vi "Main.vi"(7 "sweep rate, /min":dbl=0.2, 8 "sweep to:":dbl=4.0, 9 "sweep":T8(radio)=enum."2636a_smub") -> ()   [LabVIEW 2021] (continued)
                        n662 = property on="data_caption" class="Str"("Value"=w727) -> ()  [unwired: 2 in, 2 out]
                      }
                      frame #26 {
                        # "measure time"
                        n663 = local read "measure time"() -> (w747:bool)
                        n664 = property on="Figure_axis" class="Arr (strict)"() -> ("Value"=w744:string[])  [unwired: 2 in, 2 out]
                        n665 = property on="data_caption" class="Str"() -> ("Value"=w746:string)  [unwired: 2 in, 2 out]
                        n666 = case shown="True" w747 {
                          tunnel: w746 -> [w749 w755]
                          tunnel: [w749 w754] -> w745
                          tunnel: w744 -> [w748 w752]
                          tunnel: [w748 w750] -> w743
                          frame False {
                            # "not measuring time"
                          }
                          frame True {
                            w751 = "time"
                            # "measuring time"
                            n667 = Build Array (concatenate)(w752, w751) -> (w750:string[])
                            n668 = Concatenate Strings(w755, w751, "\t") -> (w754:string)
                          }
                        }
                        n669 = property on="Figure_axis" class="Arr (strict)"("Value"=w743) -> ()  [unwired: 2 in, 2 out]
                        n670 = property on="data_caption" class="Str"("Value"=w745) -> ()  [unwired: 2 in, 2 out]
                      }
                      frame #27 {
                        # "Measure magnetic field on Teslatron_iPS"
                        n671 = local read "MagnetField"() -> (w760:bool)
                        n672 = property on="Figure_axis" class="Arr (strict)"() -> ("Value"=w757:string[])  [unwired: 2 in, 2 out]
                        n673 = property on="data_caption" class="Str"() -> ("Value"=w759:string)  [unwired: 2 in, 2 out]
                        n674 = case shown="True" w760 {
                          tunnel: w759 -> [w762 w768]
                          tunnel: [w762 w767] -> w758
                          tunnel: w757 -> [w761 w765]
                          tunnel: [w761 w763] -> w756
                          frame False {
                            # "do not Measure magnetic field on IPS120-0"
                          }
                          frame True {
                            w764 = "MagnetField"
                            # "Measure magnetic field on Teslatron_iPS_Field"
                            n675 = Build Array (concatenate)(w765, w764) -> (w763:string[])
                            n676 = Concatenate Strings(w768, w764, "\t") -> (w767:string)
                          }
                        }
                        n677 = property on="Figure_axis" class="Arr (strict)"("Value"=w756) -> ()  [unwired: 2 in, 2 out]
                        n678 = property on="data_caption" class="Str"("Value"=w758) -> ()  [unwired: 2 in, 2 out]
                      }
                      frame #28 {
                        # "Measure magnetic Temp on Teslatron_iPS"
                        n679 = property on="Magnet_T" class="Bool (strict)"() -> ("Value"=w769:bool)  [unwired: 2 in, 2 out]
                        n680 = property on="Figure_axis" class="Arr (strict)"() -> ("Value"=w771:string[])  [unwired: 2 in, 2 out]
                        n681 = property on="data_caption" class="Str"() -> ("Value"=w773:string)  [unwired: 2 in, 2 out]
                        n682 = case shown="True" w769 {
                          tunnel: w773 -> [w775 w781]
                          tunnel: [w775 w780] -> w772
                          tunnel: w771 -> [w774 w778]
                          tunnel: [w774 w776] -> w770
                          frame False {
                            # "do not Measure magnetic field on IPS120-0"
                          }
                          frame True {
                            w777 = "Magnet_Temp"
                            # "Measure magnetic field on Teslatron_iPS_Field"
                            n683 = Build Array (concatenate)(w778, w777) -> (w776:string[])
                            n684 = Concatenate Strings(w781, w777, "\t") -> (w780:string)
                          }
                        }
                        n685 = property on="Figure_axis" class="Arr (strict)"("Value"=w770) -> ()  [unwired: 2 in, 2 out]
                        n686 = property on="data_caption" class="Str"("Value"=w772) -> ()  [unwired: 2 in, 2 out]
                      }
                      frame #29 {
                        # "Measure SH_T on Teslatron_iPS"
                        n687 = property on="PT1" class="Bool (strict)"() -> ("Value"=w782:bool)  [unwired: 2 in, 2 out]
                        n688 = property on="Figure_axis" class="Arr (strict)"() -> ("Value"=w784:string[])  [unwired: 2 in, 2 out]
                        n689 = property on="data_caption" class="Str"() -> ("Value"=w786:string)  [unwired: 2 in, 2 out]
                        n690 = case shown="True" w782 {
                          tunnel: w786 -> [w788 w794]
                          tunnel: [w788 w793] -> w785
                          tunnel: w784 -> [w787 w791]
                          tunnel: [w787 w789] -> w783
                          frame False {
                            # "do not Measure magnetic field on IPS120-0"
                          }
                          frame True {
                            w790 = "PT1_Temp"
                            # "Measure magnetic field on Teslatron_iPS_Field"
                            n691 = Build Array (concatenate)(w791, w790) -> (w789:string[])
                            n692 = Concatenate Strings(w794, w790, "\t") -> (w793:string)
                          }
                        }
                        n693 = property on="Figure_axis" class="Arr (strict)"("Value"=w783) -> ()  [unwired: 2 in, 2 out]
                        n694 = property on="data_caption" class="Str"("Value"=w785) -> ()  [unwired: 2 in, 2 out]
                      }
                      frame #30 {
                        # "Measure magnetic field on Teslatron_iPS"
                        n695 = property on="MC_RuO2" class="Bool (strict)"() -> ("Value"=w795:bool)  [unwired: 2 in, 2 out]
                        n696 = property on="Figure_axis" class="Arr (strict)"() -> ("Value"=w797:string[])  [unwired: 2 in, 2 out]
                        n697 = property on="data_caption" class="Str"() -> ("Value"=w799:string)  [unwired: 2 in, 2 out]
                        n698 = case shown="True" w795 {
                          tunnel: w799 -> [w801 w807]
                          tunnel: [w801 w806] -> w798
                          tunnel: w797 -> [w800 w804]
                          tunnel: [w800 w802] -> w796
                          frame False {
                            # "not measure 2461 voltage (2461_meas_v)"
                          }
                          frame True {
                            w803 = "MC_RuO2_Temp"
                            n699 = Build Array (concatenate)(w804, w803) -> (w802:string[])
                            n700 = Concatenate Strings(w807, w803, "\t") -> (w806:string)
                          }
                        }
                        n701 = property on="Figure_axis" class="Arr (strict)"("Value"=w796) -> ()  [unwired: 2 in, 2 out]
                        n702 = property on="data_caption" class="Str"("Value"=w798) -> ()  [unwired: 2 in, 2 out]
                      }
                      frame #31 {
                        # "Measure magnetic field on Teslatron_iPS"
                        n703 = property on="Still" class="Bool (strict)"() -> ("Value"=w808:bool)  [unwired: 2 in, 2 out]
                        n704 = property on="Figure_axis" class="Arr (strict)"() -> ("Value"=w810:string[])  [unwired: 2 in, 2 out]
                        n705 = property on="data_caption" class="Str"() -> ("Value"=w812:string)  [unwired: 2 in, 2 out]
                        n706 = case shown="True" w808 {
                          tunnel: w812 -> [w814 w820]
                          tunnel: [w814 w819] -> w811
                          tunnel: w810 -> [w813 w817]
                          tunnel: [w813 w815] -> w809
                          frame False {
                            # "not measure 2461 voltage (2461_meas_v)"
                          }
                          frame True {
                            w816 = "Still_Temp"
                            n707 = Build Array (concatenate)(w817, w816) -> (w815:string[])
                            n708 = Concatenate Strings(w820, w816, "\t") -> (w819:string)
                          }
                        }
                        n709 = property on="Figure_axis" class="Arr (strict)"("Value"=w809) -> ()  [unwired: 2 in, 2 out]
                        n710 = property on="data_caption" class="Str"("Value"=w811) -> ()  [unwired: 2 in, 2 out]
                      }
                      frame #32 {
                        # "Measure magnetic field on Teslatron_iPS"
                        n711 = property on="Cold_Plate" class="Bool (strict)"() -> ("Value"=w821:bool)  [unwired: 2 in, 2 out]
                        n712 = property on="Figure_axis" class="Arr (strict)"() -> ("Value"=w823:string[])  [unwired: 2 in, 2 out]
                        n713 = property on="data_caption" class="Str"() -> ("Value"=w825:string)  [unwired: 2 in, 2 out]
                        n714 = case shown="True" w821 {
                          tunnel: w825 -> [w827 w833]
                          tunnel: [w827 w832] -> w824
                          tunnel: w823 -> [w826 w830]
                          tunnel: [w826 w828] -> w822
                          frame False {
                            # "not measure 2461 voltage (2461_meas_v)"
                          }
                          frame True {
                            w829 = "Cold_Plate_Temp"
                            n715 = Build Array (concatenate)(w830, w829) -> (w828:string[])
                            n716 = Concatenate Strings(w833, w829, "\t") -> (w832:string)
                          }
                        }
                        n717 = property on="Figure_axis" class="Arr (strict)"("Value"=w822) -> ()  [unwired: 2 in, 2 out]
                        n718 = property on="data_caption" class="Str"("Value"=w824) -> ()  [unwired: 2 in, 2 out]
                      }
                      frame #33 {
                        # "Measure magnetic field on Teslatron_iPS"
                        n719 = property on="PT2" class="Bool (strict)"() -> ("Value"=w834:bool)  [unwired: 2 in, 2 out]
                        n720 = property on="Figure_axis" class="Arr (strict)"() -> ("Value"=w836:string[])  [unwired: 2 in, 2 out]
                        n721 = property on="data_caption" class="Str"() -> ("Value"=w838:string)  [unwired: 2 in, 2 out]
                        n722 = case shown="True" w834 {
                          tunnel: w838 -> [w840 w846]
                          tunnel: [w840 w845] -> w837
                          tunnel: w836 -> [w839 w843]
                          tunnel: [w839 w841] -> w835
                          frame False {
                            # "not measure 2461 voltage (2461_meas_v)"
                          }
                          frame True {
                            w842 = "PT2_Temp"
                            n723 = Build Array (concatenate)(w843, w842) -> (w841:string[])
                            n724 = Concatenate Strings(w846, w842, "\t") -> (w845:string)
                          }
                        }
                        n725 = property on="Figure_axis" class="Arr (strict)"("Value"=w835) -> ()  [unwired: 2 in, 2 out]
                        n726 = property on="data_caption" class="Str"("Value"=w837) -> ()  [unwired: 2 in, 2 out]
                      }
                      frame #34 {
                        # "Measure magnetic field on Teslatron_iPS"
                        n727 = property on="MC_Cernox" class="Bool (strict)"() -> ("Value"=w847:bool)  [unwired: 2 in, 2 out]
                        n728 = property on="Figure_axis" class="Arr (strict)"() -> ("Value"=w849:string[])  [unwired: 2 in, 2 out]
                        n729 = property on="data_caption" class="Str"() -> ("Value"=w851:string)  [unwired: 2 in, 2 out]
                        n730 = case shown="True" w847 {
                          tunnel: w851 -> [w853 w859]
                          tunnel: [w853 w858] -> w850
                          tunnel: w849 -> [w852 w856]
                          tunnel: [w852 w854] -> w848
                          frame False {
                            # "not measure 2461 voltage (2461_meas_v)"
                          }
                          frame True {
                            w855 = "MC_Cernox_Temp"
                            n731 = Build Array (concatenate)(w856, w855) -> (w854:string[])
                            n732 = Concatenate Strings(w859, w855, "\t") -> (w858:string)
                          }
                        }
                        n733 = property on="Figure_axis" class="Arr (strict)"("Value"=w848) -> ()  [unwired: 2 in, 2 out]
                        n734 = property on="data_caption" class="Str"("Value"=w850) -> ()  [unwired: 2 in, 2 out]
                      }
                      frame #35 {
                        # "Measure magnetic field on Teslatron_iPS"
                        n735 = property on="MFLI1_AuxOut0" class="Bool (strict)"() -> ("Value"=w860:bool)  [unwired: 2 in, 2 out]
                        n736 = property on="Figure_axis" class="Arr (strict)"() -> ("Value"=w862:string[])  [unwired: 2 in, 2 out]
                        n737 = property on="data_caption" class="Str"() -> ("Value"=w864:string)  [unwired: 2 in, 2 out]
                        n738 = case shown="True" w860 {
                          tunnel: w864 -> [w866 w872]
                          tunnel: [w866 w871] -> w863
                          tunnel: w862 -> [w865 w869]
                          tunnel: [w865 w867] -> w861
                          frame False {
                            # "not measure 2461 voltage (2461_meas_v)"
                          }
                          frame True {
                            w868 = "V_Sweep_AuxOut0"
                            n739 = Build Array (concatenate)(w869, w868) -> (w867:string[])
                            n740 = Concatenate Strings(w872, w868, "\t") -> (w871:string)
                          }
                        }
                        n741 = property on="Figure_axis" class="Arr (strict)"("Value"=w861) -> ()  [unwired: 2 in, 2 out]
                        n742 = property on="data_caption" class="Str"("Value"=w863) -> ()  [unwired: 2 in, 2 out]
                      }
                    }
                  }
                  frame #2 {
                    # "0 = SR830_1_ip\n1 = SR830_1_oop\n2 = SR830_2_ip\n3 = SR830_2_oop\n4 = SR830_3_ip\n5 = SR830_3_oop\n6 = SR830_4_ip \n7 = SR830_4_oop \n8 = SR830_5_ip \n9 = SR830_5_oop \n10= 2400_1_v \n11= 2400_1_i \n12 = 2400_2_v\n13 = 2400_2_i \n14 = 2400_3_v \n15 = 2400_3_i \n16 = 2182A_1_ch1 \n17 = 2182A_1_ch2 \n18 = 2182A_2_ch1 \n19 = 2182A_2_ch2\n20 = 2182A_3_ch1 \n21 = 2182A_3_ch2 \n22 = 2182A_4_ch1 \n23 = 2182A_4_ch2 \n24 = 2636A_smua_v \n25 = 2636A_smua_i \n26 = 2636A_smub_v \n27 = 2636A_smub_i \n28 = time\n29 = iPS_Field\n30 = iPS_Magnet_T\n31 = iPS__SH_T\n32 = iTC _sample_T\n33 = iTC _VTI_T\n34 = iTC _PT1_T\n35 = iTC _PT2_T\n36 = iTC _VTI_P\n37 = 2461_meas_v\n38= 2461_meas_i\n39= Step_Value\n40= HyperLoop_Step\n41= SuperHyper_Step"
                    n743 = stacked-sequence {
                      frame #0 {
                        w877 = dbl[] []  # Empty array for data
                        # "clear data array before each measurement cycle"
                        n744 = property on="data" class="Arr (strict)"("Value"=w877) -> (error out=w876:errorcluster)  [unwired: 2 in, 1 out]
                        n745 = property on="Sweep Channel" class="DigNum (strict)"() -> ("Value"=w873:dbl)  [unwired: 2 in, 2 out]
                        n746 = property on="data" class="Arr (strict)"(error in=w876) -> ("Value"=w875:dbl[])  [unwired: 1 in, 2 out]
                        n747 = Build Array (concatenate)(w875, w873) -> (w874:dbl[])
                        n748 = property on="data" class="Arr (strict)"("Value"=w874) -> ()  [unwired: 2 in, 2 out]
                      }
                      frame #1 {
                        n749 = stacked-sequence "measurement sequence" {
                          frame #0 {
                            # "check if in-phase\nsignal on lock-in 1 \nis to be measured"
                            n750 = property on="data" class="Arr (strict)"() -> ("Value"=w879:dbl[])  [unwired: 2 in, 2 out]
                            n751 = local read "SR830 1 ip"() -> (w878:bool)
                            n752 = case shown="True" w878 {
                              tunnel: w879 -> [w881 w890]
                              tunnel: [w881 w889] -> w880
                              frame False {
                                # "we are not measuring in phase signal on lock-in 1 (SR830_1_ip)"
                              }
                              frame True {
                                # "we are  measuring lock-in 1, in phase (SR830_1_ip)"
                                n753 = local read "SR830 1 addr"() -> (w883:u8)
                                n754 = Number To Decimal String(number=w883) -> (decimal integer string=w882:string)  [unwired: 1 in]
                                n755 = GPIB Write(0:w882, 1:"OUTR?1") -> (6:w888:errorcluster)  [unwired: 3 in, 1 out]
                                n756 = GPIB Read(0:w882, 1:3200, 3:w888) -> (5:w886:string)  [unwired: 2 in, 2 out]
                                n757 = Fract/Exp String To Number(string=w886) -> (number=w885:dbl)  [unwired: 3 in, 1 out]
                                n758 = Build Array (concatenate)(w890, w885) -> (w889:dbl[])
                              }
                            }
                            n759 = property on="data" class="Arr (strict)"("Value"=w880) -> ()  [unwired: 2 in, 2 out]
                          }
                          frame #1 {
                            # "check if out-of-phase\nsignal on lock-in 1 \nis to be measured"
                            n760 = property on="data" class="Arr (strict)"() -> ("Value"=w892:dbl[])  [unwired: 2 in, 2 out]
                            n761 = local read "SR830 1 oop"() -> (w891:bool)
                            n762 = case shown="True" w891 {
                              tunnel: w892 -> [w894 w903]
                              tunnel: [w894 w902] -> w893
                              frame False {
                                # "we are not measuring out of phase signal on lock-in 1 (SR830_1_oop)"
                              }
                              frame True {
                                # "we are  measuring lock-in 1, out of phase (SR830_1_oop)"
                                n763 = local read "SR830 1 addr"() -> (w896:u8)
                                n764 = Number To Decimal String(number=w896) -> (decimal integer string=w895:string)  [unwired: 1 in]
                                n765 = GPIB Write(0:w895, 1:"OUTR?2") -> (6:w901:errorcluster)  [unwired: 3 in, 1 out]
                                n766 = GPIB Read(0:w895, 1:3200, 3:w901) -> (5:w899:string)  [unwired: 2 in, 2 out]
                                n767 = Fract/Exp String To Number(string=w899) -> (number=w898:dbl)  [unwired: 3 in, 1 out]
                                n768 = Build Array (concatenate)(w903, w898) -> (w902:dbl[])
                              }
                            }
                            n769 = property on="data" class="Arr (strict)"("Value"=w893) -> ()  [unwired: 2 in, 2 out]
                          }
                          frame #2 {
                            # "check if in-phase\nsignal on lock-in 2 \nis to be measured"
                            n770 = property on="data" class="Arr (strict)"() -> ("Value"=w905:dbl[])  [unwired: 2 in, 2 out]
                            n771 = local read "SR830 2 ip"() -> (w904:bool)
                            n772 = case shown="True" w904 {
                              tunnel: w905 -> [w907 w916]
                              tunnel: [w907 w915] -> w906
                              frame False {
                                # "we are not measuring in phase signal on lock-in 2 (SR830_2_ip)"
                              }
                              frame True {
                                # "we are  measuring lock-in 2, in phase (SR830_2_ip)"
                                n773 = local read "SR830 2 addr"() -> (w909:u8)
                                n774 = Number To Decimal String(number=w909) -> (decimal integer string=w908:string)  [unwired: 1 in]
                                n775 = GPIB Write(0:w908, 1:"OUTP?1") -> (6:w914:errorcluster)  [unwired: 3 in, 1 out]
                                n776 = GPIB Read(0:w908, 1:3200, 3:w914) -> (5:w912:string)  [unwired: 2 in, 2 out]
                                n777 = Fract/Exp String To Number(string=w912) -> (number=w911:dbl)  [unwired: 3 in, 1 out]
                                n778 = Build Array (concatenate)(w916, w911) -> (w915:dbl[])
                              }
                            }
                            n779 = property on="data" class="Arr (strict)"("Value"=w906) -> ()  [unwired: 2 in, 2 out]
                          }
                          frame #3 {
                            # "check if out-of-phase\nsignal on lock-in 2 \nis to be measured"
                            n780 = property on="data" class="Arr (strict)"() -> ("Value"=w918:dbl[])  [unwired: 2 in, 2 out]
                            n781 = local read "SR830 2 oop"() -> (w917:bool)
                            n782 = case shown="True" w917 {
                              tunnel: w918 -> [w920 w929]
                              tunnel: [w920 w928] -> w919
                              frame False {
                                # "we are not measuring out of phase signal on lock-in 2 (SR830_2_oop)"
                              }
                              frame True {
                                # "we are  measuring lock-in 2, out of phase (SR830_2_oop)"
                                n783 = local read "SR830 2 addr"() -> (w922:u8)
                                n784 = Number To Decimal String(number=w922) -> (decimal integer string=w921:string)  [unwired: 1 in]
                                n785 = GPIB Write(0:w921, 1:"OUTP?2") -> (6:w927:errorcluster)  [unwired: 3 in, 1 out]
                                n786 = GPIB Read(0:w921, 1:3200, 3:w927) -> (5:w925:string)  [unwired: 2 in, 2 out]
                                n787 = Fract/Exp String To Number(string=w925) -> (number=w924:dbl)  [unwired: 3 in, 1 out]
                                n788 = Build Array (concatenate)(w929, w924) -> (w928:dbl[])
                              }
                            }
                            n789 = property on="data" class="Arr (strict)"("Value"=w919) -> ()  [unwired: 2 in, 2 out]
                          }
                          frame #4 {
                            # "check if in-phase\nsignal on lock-in 3 \nis to be measured"
                            n790 = property on="data" class="Arr (strict)"() -> ("Value"=w931:dbl[])  [unwired: 2 in, 2 out]
                            n791 = local read "SR830 3 ip"() -> (w930:bool)
                            n792 = case shown="True" w930 {
                              tunnel: w931 -> [w933 w942]
                              tunnel: [w933 w941] -> w932
                              frame False {
                                # "we are not measuring in phase signal on lock-in 3 (SR830_3_ip)"
                              }
                              frame True {
                                # "we are  measuring lock-in 3, in phase (SR830_3_ip)"
                                n793 = local read "SR830 3 addr"() -> (w935:u8)
                                n794 = Number To Decimal String(number=w935) -> (decimal integer string=w934:string)  [unwired: 1 in]
                                n795 = GPIB Write(0:w934, 1:"OUTP?1") -> (6:w940:errorcluster)  [unwired: 3 in, 1 out]
                                n796 = GPIB Read(0:w934, 1:3200, 3:w940) -> (5:w938:string)  [unwired: 2 in, 2 out]
                                n797 = Fract/Exp String To Number(string=w938) -> (number=w937:dbl)  [unwired: 3 in, 1 out]
                                n798 = Build Array (concatenate)(w942, w937) -> (w941:dbl[])
                              }
                            }
                            n799 = property on="data" class="Arr (strict)"("Value"=w932) -> ()  [unwired: 2 in, 2 out]
                          }
                          frame #5 {
                            # "check if out-of-phase\nsignal on lock-in 3 \nis to be measured"
                            n800 = property on="data" class="Arr (strict)"() -> ("Value"=w944:dbl[])  [unwired: 2 in, 2 out]
                            n801 = local read "SR830 3 oop"() -> (w943:bool)
                            n802 = case shown="True" w943 {
                              tunnel: w944 -> [w946 w955]
                              tunnel: [w946 w954] -> w945
                              frame False {
                                # "we are not measuring out of phase signal on lock-in 3 (SR830_3_oop)"
                              }
                              frame True {
                                # "we are  measuring lock-in 3, out of phase (SR830_3_oop)"
                                n803 = local read "SR830 3 addr"() -> (w948:u8)
                                n804 = Number To Decimal String(number=w948) -> (decimal integer string=w947:string)  [unwired: 1 in]
                                n805 = GPIB Write(0:w947, 1:"OUTP?2") -> (6:w953:errorcluster)  [unwired: 3 in, 1 out]
                                n806 = GPIB Read(0:w947, 1:3200, 3:w953) -> (5:w951:string)  [unwired: 2 in, 2 out]
                                n807 = Fract/Exp String To Number(string=w951) -> (number=w950:dbl)  [unwired: 3 in, 1 out]
                                n808 = Build Array (concatenate)(w955, w950) -> (w954:dbl[])
                              }
                            }
                            n809 = property on="data" class="Arr (strict)"("Value"=w945) -> ()  [unwired: 2 in, 2 out]
                          }
                          frame #6 {
                            # "check if in-phase\nsignal on lock-in 4 \nis to be measured"
                            n810 = property on="data" class="Arr (strict)"() -> ("Value"=w957:dbl[])  [unwired: 2 in, 2 out]
                            n811 = local read "SR830 4 ip"() -> (w956:bool)
                            n812 = case shown="True" w956 {
                              tunnel: w957 -> [w959 w968]
                              tunnel: [w959 w967] -> w958
                              frame False {
                                # "we are not measuring in phase signal on lock-in 4 (SR830_4_ip)"
                              }
                              frame True {
                                # "we are  measuring lock-in 4, in phase (SR830_4_ip)"
                                n813 = local read "SR830 4 addr"() -> (w961:u8)
                                n814 = Number To Decimal String(number=w961) -> (decimal integer string=w960:string)  [unwired: 1 in]
                                n815 = GPIB Write(0:w960, 1:"OUTP?1") -> (6:w966:errorcluster)  [unwired: 3 in, 1 out]
                                n816 = GPIB Read(0:w960, 1:3200, 3:w966) -> (5:w964:string)  [unwired: 2 in, 2 out]
                                n817 = Fract/Exp String To Number(string=w964) -> (number=w963:dbl)  [unwired: 3 in, 1 out]
                                n818 = Build Array (concatenate)(w968, w963) -> (w967:dbl[])
                              }
                            }
                            n819 = property on="data" class="Arr (strict)"("Value"=w958) -> ()  [unwired: 2 in, 2 out]
                          }
                          frame #7 {
                            # "check if out-of-phase\nsignal on lock-in 4 \nis to be measured"
                            n820 = property on="data" class="Arr (strict)"() -> ("Value"=w970:dbl[])  [unwired: 2 in, 2 out]
                            n821 = local read "SR830 4 oop"() -> (w969:bool)
                            n822 = case shown="True" w969 {
                              tunnel: w970 -> [w972 w981]
                              tunnel: [w972 w980] -> w971
                              frame False {
                                # "we are not measuring out of phase signal on lock-in 4 (SR830_4_oop)"
                              }
                              frame True {
                                # "we are  measuring lock-in 4, out of phase (SR830_4_oop)"
                                n823 = local read "SR830 4 addr"() -> (w974:u8)
                                n824 = Number To Decimal String(number=w974) -> (decimal integer string=w973:string)  [unwired: 1 in]
                                n825 = GPIB Write(0:w973, 1:"OUTP?2") -> (6:w979:errorcluster)  [unwired: 3 in, 1 out]
                                n826 = GPIB Read(0:w973, 1:3200, 3:w979) -> (5:w977:string)  [unwired: 2 in, 2 out]
                                n827 = Fract/Exp String To Number(string=w977) -> (number=w976:dbl)  [unwired: 3 in, 1 out]
                                n828 = Build Array (concatenate)(w981, w976) -> (w980:dbl[])
                              }
                            }
                            n829 = property on="data" class="Arr (strict)"("Value"=w971) -> ()  [unwired: 2 in, 2 out]
                          }
                          frame #8 {
                            n830 = property on="data" class="Arr (strict)"() -> ("Value"=w983:dbl[])  [unwired: 2 in, 2 out]
                            n831 = local read "SR830 5 ip"() -> (w982:bool)
                            n832 = case shown="True" w982 {
                              tunnel: w983 -> [w985 w994]
                              tunnel: [w985 w993] -> w984
                              frame False {
                              }
                              frame True {
                                n833 = local read "SR830 5 addr"() -> (w987:u8)
                                n834 = Number To Decimal String(number=w987) -> (decimal integer string=w986:string)  [unwired: 1 in]
                                n835 = GPIB Write(0:w986, 1:"OUTP?1") -> (6:w992:errorcluster)  [unwired: 3 in, 1 out]
                                n836 = GPIB Read(0:w986, 1:3200, 3:w992) -> (5:w990:string)  [unwired: 2 in, 2 out]
                                n837 = Fract/Exp String To Number(string=w990) -> (number=w989:dbl)  [unwired: 3 in, 1 out]
                                n838 = Build Array (concatenate)(w994, w989) -> (w993:dbl[])
                              }
                            }
                            n839 = property on="data" class="Arr (strict)"("Value"=w984) -> ()  [unwired: 2 in, 2 out]
                          }
                          frame #9 {
                            n840 = property on="data" class="Arr (strict)"() -> ("Value"=w996:dbl[])  [unwired: 2 in, 2 out]
                            n841 = local read "SR830 5 oop"() -> (w995:bool)
                            n842 = case shown="True" w995 {
                              tunnel: w996 -> [w998 w1007]
                              tunnel: [w998 w1006] -> w997
                              frame False {
                                # "we are not measuring out of phase signal on lock-in 4 (SR830_4_oop)"
                              }
                              frame True {
                                n843 = local read "SR830 5 addr"() -> (w1000:u8)
                                n844 = Number To Decimal String(number=w1000) -> (decimal integer string=w999:string)  [unwired: 1 in]
                                n845 = GPIB Write(0:w999, 1:"OUTP?2") -> (6:w1005:errorcluster)  [unwired: 3 in, 1 out]
                                n846 = GPIB Read(0:w999, 1:3200, 3:w1005) -> (5:w1003:string)  [unwired: 2 in, 2 out]
                                n847 = Fract/Exp String To Number(string=w1003) -> (number=w1002:dbl)  [unwired: 3 in, 1 out]
                                n848 = Build Array (concatenate)(w1007, w1002) -> (w1006:dbl[])
                              }
                            }
                            n849 = property on="data" class="Arr (strict)"("Value"=w997) -> ()  [unwired: 2 in, 2 out]
                          }
                          frame #10 {
                            # "check if voltage \non 2400 SouceMeter 1\nis to be measured"
                            n850 = property on="data" class="Arr (strict)"() -> ("Value"=w1009:dbl[])  [unwired: 2 in, 2 out]
                            n851 = local read "2400 1 meas v"() -> (w1008:bool)
                            n852 = case shown="True" w1008 {
                              tunnel: w1009 -> [w1011 w1022]
                              tunnel: [w1011 w1021] -> w1010
                              frame False {
                                # "we are not measuring 2400 1, voltage (2400_1_v)"
                              }
                              frame True {
                                # "we are  measuring 2400 1, voltage (2400_1_v)"
                                n853 = local read "2400 1 addr"() -> (w1016:u8)
                                n854 = Number To Decimal String(number=w1016) -> (decimal integer string=w1015:string)  [unwired: 1 in]
                                n855 = GPIB Write(0:w1015, 1:":READ?") -> (6:w1020:errorcluster)  [unwired: 3 in, 1 out]
                                n856 = GPIB Read(0:w1015, 1:3200, 3:w1020) -> (5:w1013:string)  [unwired: 2 in, 2 out]
                                n857 = String Subset(string=w1013, length (rest)=13) -> (substring=w1012:string)  [unwired: 1 in]
                                n858 = Fract/Exp String To Number(string=w1012) -> (number=w1018:dbl)  [unwired: 3 in, 1 out]
                                n859 = Build Array (concatenate)(w1022, w1018) -> (w1021:dbl[])
                              }
                            }
                            n860 = property on="data" class="Arr (strict)"("Value"=w1010) -> ()  [unwired: 2 in, 2 out]
                          }
                          frame #11 {
                            # "check if current \non 2400 SouceMeter 1\nis to be measured"
                            n861 = property on="data" class="Arr (strict)"() -> ("Value"=w1024:dbl[])  [unwired: 2 in, 2 out]
                            n862 = local read "2400 1 meas i"() -> (w1023:bool)
                            n863 = case shown="True" w1023 {
                              tunnel: w1024 -> [w1026 w1038]
                              tunnel: [w1026 w1037] -> w1025
                              frame False {
                                # "we are not measuring 2400 1, current (2400_1_i)"
                              }
                              frame True {
                                # "we are  measuring 2400 1, current (2400_1_i)"
                                n864 = local read "2400 1 addr"() -> (w1032:u8)
                                n865 = Number To Decimal String(number=w1032) -> (decimal integer string=w1031:string)  [unwired: 1 in]
                                n866 = GPIB Write(0:w1031, 1:":READ?") -> (6:w1036:errorcluster)  [unwired: 3 in, 1 out]
                                n867 = GPIB Read(0:w1031, 1:3200, 3:w1036) -> (5:w1029:string)  [unwired: 2 in, 2 out]
                                n868 = String Subset(string=w1029, offset (0)=14, length (rest)=13) -> (substring=w1028:string)
                                n869 = Fract/Exp String To Number(string=w1028) -> (number=w1034:dbl)  [unwired: 3 in, 1 out]
                                n870 = Build Array (concatenate)(w1038, w1034) -> (w1037:dbl[])
                              }
                            }
                            n871 = property on="data" class="Arr (strict)"("Value"=w1025) -> ()  [unwired: 2 in, 2 out]
                          }
                          frame #12 {
                            # "check if voltage \non 2400 SouceMeter 2\nis to be measured"
                            n872 = property on="data" class="Arr (strict)"() -> ("Value"=w1040:dbl[])  [unwired: 2 in, 2 out]
                            n873 = local read "2400 2 meas v"() -> (w1039:bool)
                            n874 = case shown="True" w1039 {
                              tunnel: w1040 -> [w1042 w1053]
                              tunnel: [w1042 w1052] -> w1041
                              frame False {
                                # "we are not measuring 2400 2, voltage (2400_2_v)"
                              }
                              frame True {
                                # "we are  measuring 2400 2, voltage (2400_2_v)"
                                n875 = local read "2400 2 addr"() -> (w1047:u8)
                                n876 = Number To Decimal String(number=w1047) -> (decimal integer string=w1046:string)  [unwired: 1 in]
                                n877 = GPIB Write(0:w1046, 1:":READ?") -> (6:w1051:errorcluster)  [unwired: 3 in, 1 out]
                                n878 = GPIB Read(0:w1046, 1:3200, 3:w1051) -> (5:w1044:string)  [unwired: 2 in, 2 out]
                                n879 = String Subset(string=w1044, length (rest)=13) -> (substring=w1043:string)  [unwired: 1 in]
                                n880 = Fract/Exp String To Number(string=w1043) -> (number=w1049:dbl)  [unwired: 3 in, 1 out]
                                n881 = Build Array (concatenate)(w1053, w1049) -> (w1052:dbl[])
                              }
                            }
                            n882 = property on="data" class="Arr (strict)"("Value"=w1041) -> ()  [unwired: 2 in, 2 out]
                          }
                          frame #13 {
                            # "check if current \non 2400 SouceMeter 2\nis to be measured"
                            n883 = property on="data" class="Arr (strict)"() -> ("Value"=w1055:dbl[])  [unwired: 2 in, 2 out]
                            n884 = local read "2400 2 meas i"() -> (w1054:bool)
                            n885 = case shown="True" w1054 {
                              tunnel: w1055 -> [w1057 w1069]
                              tunnel: [w1057 w1068] -> w1056
                              frame False {
                                # "we are not measuring 2400 2, current (2400_2_i)"
                              }
                              frame True {
                                # "we are  measuring 2400 2, current (2400_2_i)"
                                n886 = local read "2400 2 addr"() -> (w1063:u8)
                                n887 = Number To Decimal String(number=w1063) -> (decimal integer string=w1062:string)  [unwired: 1 in]
                                n888 = GPIB Write(0:w1062, 1:":READ?") -> (6:w1067:errorcluster)  [unwired: 3 in, 1 out]
                                n889 = GPIB Read(0:w1062, 1:3200, 3:w1067) -> (5:w1060:string)  [unwired: 2 in, 2 out]
                                n890 = String Subset(string=w1060, offset (0)=14, length (rest)=13) -> (substring=w1059:string)
                                n891 = Fract/Exp String To Number(string=w1059) -> (number=w1065:dbl)  [unwired: 3 in, 1 out]
                                n892 = Build Array (concatenate)(w1069, w1065) -> (w1068:dbl[])
                              }
                            }
                            n893 = property on="data" class="Arr (strict)"("Value"=w1056) -> ()  [unwired: 2 in, 2 out]
                          }
                          frame #14 {
                            # "check if voltage \non 2400 SouceMeter 3\nis to be measured"
                            n894 = property on="data" class="Arr (strict)"() -> ("Value"=w1071:dbl[])  [unwired: 2 in, 2 out]
                            n895 = local read "2400 3 meas v"() -> (w1070:bool)
                            n896 = case shown="True" w1070 {
                              tunnel: w1071 -> [w1073 w1084]
                              tunnel: [w1073 w1083] -> w1072
                              frame False {
                                # "we are not measuring 2400 3, voltage (2400_3_v)"
                              }
                              frame True {
                                # "we are  measuring 2400 3, voltage (2400_3_v)"
                                n897 = local read "2400 3 addr"() -> (w1078:u8)
                                n898 = Number To Decimal String(number=w1078) -> (decimal integer string=w1077:string)  [unwired: 1 in]
                                n899 = GPIB Write(0:w1077, 1:":READ?") -> (6:w1082:errorcluster)  [unwired: 3 in, 1 out]
                                n900 = GPIB Read(0:w1077, 1:3200, 3:w1082) -> (5:w1075:string)  [unwired: 2 in, 2 out]
                                n901 = String Subset(string=w1075, length (rest)=13) -> (substring=w1074:string)  [unwired: 1 in]
                                n902 = Fract/Exp String To Number(string=w1074) -> (number=w1080:dbl)  [unwired: 3 in, 1 out]
                                n903 = Build Array (concatenate)(w1084, w1080) -> (w1083:dbl[])
                              }
                            }
                            n904 = property on="data" class="Arr (strict)"("Value"=w1072) -> ()  [unwired: 2 in, 2 out]
                          }
                          frame #15 {
                            # "check if current \non 2400 SouceMeter 3\nis to be measured"
                            n905 = property on="data" class="Arr (strict)"() -> ("Value"=w1086:dbl[])  [unwired: 2 in, 2 out]
                            n906 = local read "2400 3 meas i"() -> (w1085:bool)
                            n907 = case shown="True" w1085 {
                              tunnel: w1086 -> [w1088 w1100]
                              tunnel: [w1088 w1099] -> w1087
                              frame False {
                                # "we are not measuring 2400 3, current (2400_3_i)"
                              }
                              frame True {
                                # "we are  measuring 2400 3, current (2400_3_i)"
                                n908 = local read "2400 3 addr"() -> (w1094:u8)
                                n909 = Number To Decimal String(number=w1094) -> (decimal integer string=w1093:string)  [unwired: 1 in]
                                n910 = GPIB Write(0:w1093, 1:":READ?") -> (6:w1098:errorcluster)  [unwired: 3 in, 1 out]
                                n911 = GPIB Read(0:w1093, 1:3200, 3:w1098) -> (5:w1091:string)  [unwired: 2 in, 2 out]
                                n912 = String Subset(string=w1091, offset (0)=14, length (rest)=13) -> (substring=w1090:string)
                                n913 = Fract/Exp String To Number(string=w1090) -> (number=w1096:dbl)  [unwired: 3 in, 1 out]
                                n914 = Build Array (concatenate)(w1100, w1096) -> (w1099:dbl[])
                              }
                            }
                            n915 = property on="data" class="Arr (strict)"("Value"=w1087) -> ()  [unwired: 2 in, 2 out]
                          }
                          frame #16 {
                            # "check if 1st channel \non Keithley 2182A 1\nis to be measured"
                            n916 = property on="data" class="Arr (strict)"() -> ("Value"=w1102:dbl[])  [unwired: 2 in, 2 out]
                            n917 = local read "2182A 1 ch1"() -> (w1101:bool)
                            n918 = case shown="True" w1101 {
                              tunnel: w1102 -> [w1104 w1113]
                              tunnel: [w1104 w1112] -> w1103
                              frame False {
                                # "we are not measuring 2182A 1 channel 1 (2182A_1_ch1)"
                              }
                              frame True {
                                # "we are  measuring 2182A 1 channel 1 (2182A_1_ch1)"
                                n919 = local read "2182A 1 addr"() -> (w1107:u8)
                                n920 = Number To Decimal String(number=w1107) -> (decimal integer string=w1106:string)  [unwired: 1 in]
                                n921 = GPIB Write(0:w1106, 1:":SENSe:DATA:FRES?") -> (6:w1111:errorcluster)  [unwired: 3 in, 1 out]
                                n922 = GPIB Read(0:w1106, 1:200, 3:w1111) -> (5:w1105:string)  [unwired: 2 in, 2 out]
                                n923 = Fract/Exp String To Number(string=w1105) -> (number=w1109:dbl)  [unwired: 3 in, 1 out]
                                n924 = Build Array (concatenate)(w1113, w1109) -> (w1112:dbl[])
                              }
                            }
                            n925 = property on="data" class="Arr (strict)"("Value"=w1103) -> ()  [unwired: 2 in, 2 out]
                          }
                          frame #17 {
                            # "check if 2nd channel \non Keithley 2182A 1\nis to be measured"
                            n926 = property on="data" class="Arr (strict)"() -> ("Value"=w1115:dbl[])  [unwired: 2 in, 2 out]
                            n927 = local read "2182A 1 ch2"() -> (w1114:bool)
                            n928 = case shown="True" w1114 {
                              tunnel: w1115 -> [w1117 w1130]
                              tunnel: [w1117 w1129] -> w1116
                              frame False {
                                # "we are not measuring 2182A 1 channel 2 (2182A_1_ch2)"
                              }
                              frame True {
                                # "switching to channel 2 and then\nback to channel 1"
                                # "we are  measuring 2182A 1 channel 2 (2182A_1_ch2)"
                                n929 = local read "2182A 1 addr"() -> (w1124:u8)
                                n930 = Number To Decimal String(number=w1124) -> (decimal integer string=w1119:string)  [unwired: 1 in]
                                n931 = GPIB Write(0:w1119, 1:":SENSe:CHAN 2") -> (6:w1121:errorcluster)  [unwired: 3 in, 1 out]
                                n932 = GPIB Write(0:w1119, 1:":SENSe:DATA:FRES?", 3:w1121) -> (6:w1128:errorcluster)  [unwired: 2 in, 1 out]
                                n933 = GPIB Read(0:w1119, 1:200, 3:w1128) -> (5:w1123:string, 7:w1120:errorcluster)  [unwired: 2 in, 1 out]
                                n934 = GPIB Write(0:w1119, 1:":SENSe:CHAN 1", 3:w1120) -> ()  [unwired: 2 in, 2 out]
                                n935 = Fract/Exp String To Number(string=w1123) -> (number=w1126:dbl)  [unwired: 3 in, 1 out]
                                n936 = Build Array (concatenate)(w1130, w1126) -> (w1129:dbl[])
                              }
                            }
                            n937 = property on="data" class="Arr (strict)"("Value"=w1116) -> ()  [unwired: 2 in, 2 out]
                          }
                          frame #18 {
                            # "check if 1st channel \non Keithley 2182A 2\nis to be measured"
                            n938 = property on="data" class="Arr (strict)"() -> ("Value"=w1132:dbl[])  [unwired: 2 in, 2 out]
                            n939 = local read "2182A 2 ch1"() -> (w1131:bool)
                            n940 = case shown="False" w1131 {
                              tunnel: w1132 -> [w1134 w1143]
                              tunnel: [w1134 w1142] -> w1133
                              frame False {
                                # "we are not measuring 2182A 2 channel 1 (2182A_2_ch1)"
                              }
                              frame True {
                                # "we are  measuring 2182A 2 channel 1 (2182A_2_ch1)"
                                n941 = local read "2182A 2 addr"() -> (w1137:u8)
                                n942 = Number To Decimal String(number=w1137) -> (decimal integer string=w1136:string)  [unwired: 1 in]
                                n943 = GPIB Write(0:w1136, 1:":SENSe:DATA:FRES?") -> (6:w1141:errorcluster)  [unwired: 3 in, 1 out]
                                n944 = GPIB Read(0:w1136, 1:200, 3:w1141) -> (5:w1135:string)  [unwired: 2 in, 2 out]
                                n945 = Fract/Exp String To Number(string=w1135) -> (number=w1139:dbl)  [unwired: 3 in, 1 out]
                                n946 = Build Array (concatenate)(w1143, w1139) -> (w1142:dbl[])
                              }
                            }
                            n947 = property on="data" class="Arr (strict)"("Value"=w1133) -> ()  [unwired: 2 in, 2 out]
                          }
                          frame #19 {
                            # "check if 2nd channel \non Keithley 2182A 2\nis to be measured"
                            n948 = property on="data" class="Arr (strict)"() -> ("Value"=w1145:dbl[])  [unwired: 2 in, 2 out]
                            n949 = local read "2182A 2 ch2"() -> (w1144:bool)
                            n950 = case shown="True" w1144 {
                              tunnel: w1145 -> [w1147 w1160]
                              tunnel: [w1147 w1159] -> w1146
                              frame False {
                                # "we are not measuring 2182A 2 channel 2 (2182A_2_ch2)"
                              }
                              frame True {
                                # "switching to channel 2 and then\nback to channel 1"
                                # "we are  measuring 2182A 2 channel 2 (2182A_2_ch2)"
                                n951 = local read "2182A 2 addr"() -> (w1154:u8)
                                n952 = Number To Decimal String(number=w1154) -> (decimal integer string=w1149:string)  [unwired: 1 in]
                                n953 = GPIB Write(0:w1149, 1:":SENSe:CHAN 2") -> (6:w1151:errorcluster)  [unwired: 3 in, 1 out]
                                n954 = GPIB Write(0:w1149, 1:":SENSe:DATA:FRES?", 3:w1151) -> (6:w1158:errorcluster)  [unwired: 2 in, 1 out]
                                n955 = GPIB Read(0:w1149, 1:200, 3:w1158) -> (5:w1153:string, 7:w1150:errorcluster)  [unwired: 2 in, 1 out]
                                n956 = GPIB Write(0:w1149, 1:":SENSe:CHAN 1", 3:w1150) -> ()  [unwired: 2 in, 2 out]
                                n957 = Fract/Exp String To Number(string=w1153) -> (number=w1156:dbl)  [unwired: 3 in, 1 out]
                                n958 = Build Array (concatenate)(w1160, w1156) -> (w1159:dbl[])
                              }
                            }
                            n959 = property on="data" class="Arr (strict)"("Value"=w1146) -> ()  [unwired: 2 in, 2 out]
                          }
                          frame #20 {
                            # "check if 1st channel \non Keithley 2182A 3\nis to be measured"
                            n960 = property on="data" class="Arr (strict)"() -> ("Value"=w1162:dbl[])  [unwired: 2 in, 2 out]
                            n961 = local read "2182A 3 ch1"() -> (w1161:bool)
                            n962 = case shown="True" w1161 {
                              tunnel: w1162 -> [w1164 w1173]
                              tunnel: [w1164 w1172] -> w1163
                              frame False {
                                # "we are not measuring 2182A 3 channel 1 (2182A_3_ch1)"
                              }
                              frame True {
                                # "we are  measuring 2182A 3 channel 1 (2182A_3_ch1)"
                                n963 = local read "2182A 3 addr"() -> (w1167:u8)
                                n964 = Number To Decimal String(number=w1167) -> (decimal integer string=w1166:string)  [unwired: 1 in]
                                n965 = GPIB Write(0:w1166, 1:":SENSe:DATA:FRES?") -> (6:w1171:errorcluster)  [unwired: 3 in, 1 out]
                                n966 = GPIB Read(0:w1166, 1:200, 3:w1171) -> (5:w1165:string)  [unwired: 2 in, 2 out]
                                n967 = Fract/Exp String To Number(string=w1165) -> (number=w1169:dbl)  [unwired: 3 in, 1 out]
                                n968 = Build Array (concatenate)(w1173, w1169) -> (w1172:dbl[])
                              }
                            }
                            n969 = property on="data" class="Arr (strict)"("Value"=w1163) -> ()  [unwired: 2 in, 2 out]
                          }
                          frame #21 {
                            # "check if 2nd channel \non Keithley 2182A 3\nis to be measured"
                            n970 = property on="data" class="Arr (strict)"() -> ("Value"=w1175:dbl[])  [unwired: 2 in, 2 out]
                            n971 = local read "2182A 3 ch2"() -> (w1174:bool)
                            n972 = case shown="True" w1174 {
                              tunnel: w1175 -> [w1177 w1190]
                              tunnel: [w1177 w1189] -> w1176
                              frame False {
                                # "we are not measuring 2182A 3 channel 2 (2182A_3_ch2)"
                              }
                              frame True {
                                # "switching to channel 2 and then\nback to channel 1"
                                # "we are  measuring 2182A 3 channel 2 (2182A_3_ch2)"
                                n973 = local read "2182A 3 addr"() -> (w1184:u8)
                                n974 = Number To Decimal String(number=w1184) -> (decimal integer string=w1179:string)  [unwired: 1 in]
                                n975 = GPIB Write(0:w1179, 1:":SENSe:CHAN 2") -> (6:w1181:errorcluster)  [unwired: 3 in, 1 out]
                                n976 = GPIB Write(0:w1179, 1:":SENSe:DATA:FRES?", 3:w1181) -> (6:w1188:errorcluster)  [unwired: 2 in, 1 out]
                                n977 = GPIB Read(0:w1179, 1:200, 3:w1188) -> (5:w1183:string, 7:w1180:errorcluster)  [unwired: 2 in, 1 out]
                                n978 = GPIB Write(0:w1179, 1:":SENSe:CHAN 1", 3:w1180) -> ()  [unwired: 2 in, 2 out]
                                n979 = Fract/Exp String To Number(string=w1183) -> (number=w1186:dbl)  [unwired: 3 in, 1 out]
                                n980 = Build Array (concatenate)(w1190, w1186) -> (w1189:dbl[])
                              }
                            }
                            n981 = property on="data" class="Arr (strict)"("Value"=w1176) -> ()  [unwired: 2 in, 2 out]
                          }
                          frame #22 {
                            # "check if 1st channel \non Keithley 2182A 4\nis to be measured"
                            n982 = property on="data" class="Arr (strict)"() -> ("Value"=w1192:dbl[])  [unwired: 2 in, 2 out]
                            n983 = local read "2182A 4 ch1"() -> (w1191:bool)
                            n984 = case shown="True" w1191 {
                              tunnel: w1192 -> [w1194 w1203]
                              tunnel: [w1194 w1202] -> w1193
                              frame False {
                                # "we are not measuring 2182A 4 channel 1 (2182A_4_ch1)"
                              }
                              frame True {
                                # "we are  measuring 2182A 4 channel 1 (2182A_4_ch1)"
                                n985 = local read "2182A 4 addr"() -> (w1197:u8)
                                n986 = Number To Decimal String(number=w1197) -> (decimal integer string=w1196:string)  [unwired: 1 in]
                                n987 = GPIB Write(0:w1196, 1:":SENSe:DATA:FRES?") -> (6:w1201:errorcluster)  [unwired: 3 in, 1 out]
                                n988 = GPIB Read(0:w1196, 1:200, 3:w1201) -> (5:w1195:string)  [unwired: 2 in, 2 out]
                                n989 = Fract/Exp String To Number(string=w1195) -> (number=w1199:dbl)  [unwired: 3 in, 1 out]
                                n990 = Build Array (concatenate)(w1203, w1199) -> (w1202:dbl[])
                              }
                            }
                            n991 = property on="data" class="Arr (strict)"("Value"=w1193) -> ()  [unwired: 2 in, 2 out]
                          }
                          frame #23 {
                            # "check if 2nd channel \non Keithley 2182A 4\nis to be measured"
                            n992 = property on="data" class="Arr (strict)"() -> ("Value"=w1205:dbl[])  [unwired: 2 in, 2 out]
                            n993 = local read "2182A 4 ch2"() -> (w1204:bool)
                            n994 = case shown="False" w1204 {
                              tunnel: w1205 -> [w1207 w1220]
                              tunnel: [w1207 w1219] -> w1206
                              frame False {
                                # "we are not measuring 2182A 4 channel 2 (2182A_4_ch2)"
                              }
                              frame True {
                                # "switching to channel 2 and then\nback to channel 1"
                                # "we are  measuring 2182A 4 channel 2 (2182A_4_ch2)"
                                n995 = local read "2182A 4 addr"() -> (w1214:u8)
                                n996 = Number To Decimal String(number=w1214) -> (decimal integer string=w1209:string)  [unwired: 1 in]
                                n997 = GPIB Write(0:w1209, 1:":SENSe:CHAN 2") -> (6:w1211:errorcluster)  [unwired: 3 in, 1 out]
                                n998 = GPIB Write(0:w1209, 1:":SENSe:DATA:FRES?", 3:w1211) -> (6:w1218:errorcluster)  [unwired: 2 in, 1 out]
                                n999 = GPIB Read(0:w1209, 1:200, 3:w1218) -> (5:w1213:string, 7:w1210:errorcluster)  [unwired: 2 in, 1 out]
                                n1000 = GPIB Write(0:w1209, 1:":SENSe:CHAN 1", 3:w1210) -> ()  [unwired: 2 in, 2 out]
                                n1001 = Fract/Exp String To Number(string=w1213) -> (number=w1216:dbl)  [unwired: 3 in, 1 out]
                                n1002 = Build Array (concatenate)(w1220, w1216) -> (w1219:dbl[])
                              }
                            }
                            n1003 = property on="data" class="Arr (strict)"("Value"=w1206) -> ()  [unwired: 2 in, 2 out]
                          }
                          frame #24 {
                            # "check if voltage on\nKeithley 2636A smua\nis to be measured"
                            n1004 = local read "2636A smua meas v"() -> (w1221:bool)
                            n1005 = property on="data" class="Arr (strict)"() -> ("Value"=w1222:dbl[])  [unwired: 2 in, 2 out]
                            n1006 = case shown="True" w1221 {
                              tunnel: w1222 -> [w1224 w1230]
                              tunnel: [w1224 w1229] -> w1223
                              frame False {
                                # "we are not measuring voltage on 2636A smua (2636A_smua_v)"
